vi "Configure Serial Bus (I2S - Trigger).vi"(0 "VISA resource name":refnum<visa-resource-name>, 1 "Data Pattern (0)":string="0", 2 "Lower Threshold (-10)":i32=-10, 5 "Serial Bus Name (1: Serial Bus 1)":i32(ring)=1 items=["Serial Bus 1"=1, "Serial Bus 2"=2], 7 "Trigger Operator (0: Equal)":i32(ring) items=["Equal", "Not Equal", "Less Than", "Greater Than", "In Range", "Out Range", "Increasing", "Decreasing"], 9 "Audio Channel (0: Right Channel)":i32(ring) items=["Right Channel", "Left Channel", "Either"], 11 "error in (no error)":errorcluster, 12 "Pattern Format (0: Binary)":i32(ring) items=["Binary", "Hex", "Decimal"], 13 "Higher Threshold (10)":i32=10) -> (4 "VISA resource name out":refnum<visa-resource-name>, 15 "error out":errorcluster)   [LabVIEW 2017, in "Agilent 2000 3000 X-Series.lvlib"]
doc: "Configures the trigger settings of I2S bus.\n\nNote:\nThis VI is not supported by 1000 X Series"
uses:
  Agilent 2000 3000 X-Series.lvlib
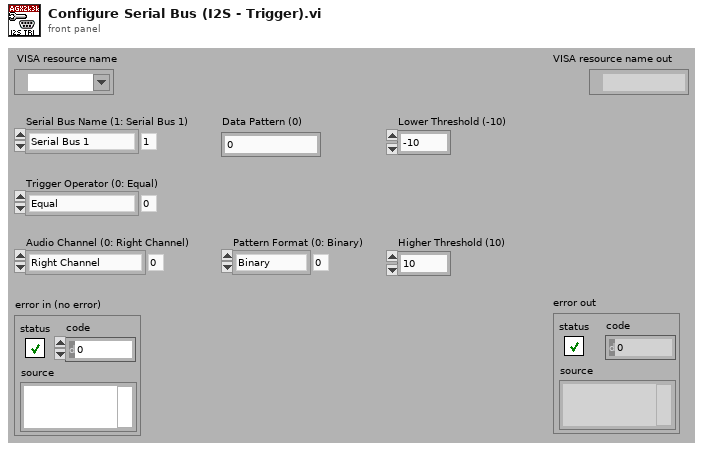
[diagram p1: front panel]
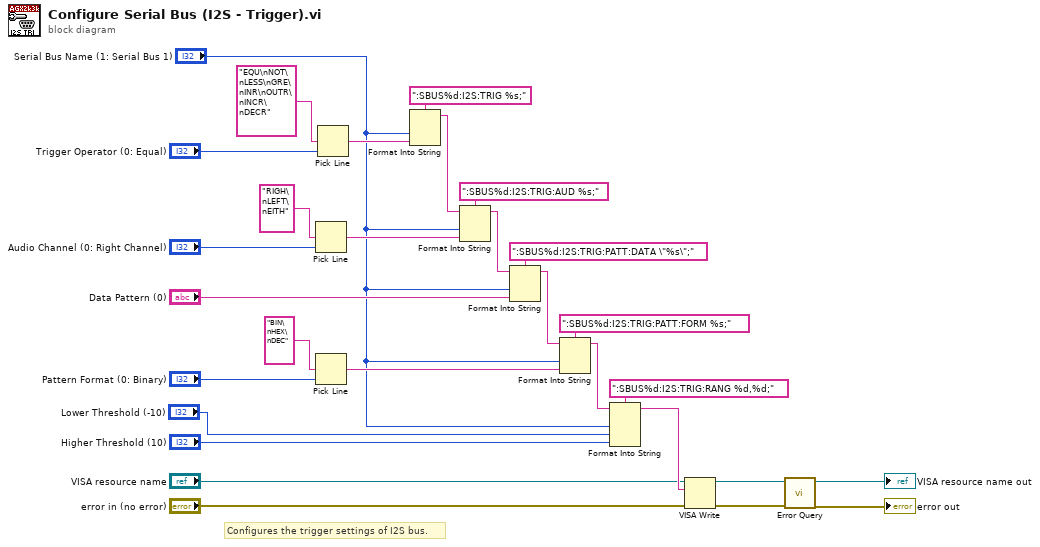
[diagram p0: block diagram]
diagram:
  # "Configures the trigger settings of I2S bus."
  n1 = Pick Line(multi-line string="RIGH\nLEFT\nEITH", line index="Audio Channel (0: Right Channel)") -> (output string=w21:string)  [unwired: 1 out]
  n2 = Pick Line(multi-line string="BIN\nHEX\nDEC", line index="Pattern Format (0: Binary)") -> (output string=w13:string)  [unwired: 1 out]
  n3 = Pick Line(multi-line string="EQU\nNOT\nLESS\nGRE\nINR\nOUTR\nINCR\nDECR", line index="Trigger Operator (0: Equal)") -> (output string=w26:string)  [unwired: 1 out]
  n4 = Format Into String(format string=":SBUS%d:I2S:TRIG %s;", "Serial Bus Name (1: Serial Bus 1)", w26) -> (resulting string=w23:string)  [unwired: 2 in, 1 out]
  n5 = Format Into String(format string=":SBUS%d:I2S:TRIG:AUD %s;", initial string=w23, "Serial Bus Name (1: Serial Bus 1)", w21) -> (resulting string=w20:string)  [unwired: 1 in, 1 out]
  n6 = Format Into String(format string=":SBUS%d:I2S:TRIG:PATT:DATA \"%s\";", initial string=w20, "Serial Bus Name (1: Serial Bus 1)", "Data Pattern (0)") -> (resulting string=w15:string)  [unwired: 1 in, 1 out]
  n7 = Format Into String(format string=":SBUS%d:I2S:TRIG:PATT:FORM %s;", initial string=w15, "Serial Bus Name (1: Serial Bus 1)", w13) -> (resulting string=w12:string)  [unwired: 1 in, 1 out]
  n8 = Format Into String(format string=":SBUS%d:I2S:TRIG:RANG %d,%d;", initial string=w12, "Serial Bus Name (1: Serial Bus 1)", "Lower Threshold (-10)", "Higher Threshold (10)") -> (resulting string=w8:string)  [unwired: 1 in, 1 out]
  n9 = VISA Write(VISA resource name="VISA resource name", write buffer=w8, error in (no error)="error in (no error)") -> (VISA resource name out=w5:refnum<visa-resource-name>, error out=w4:errorcluster)  [unwired: 1 out]
  n10 = call "Error Query.vi"("error in (no error)"=w4, "VISA resource name"=w5) -> ("error out"=→"error out":errorcluster, "VISA resource name out"=→"VISA resource name out":refnum<visa-resource-name>)  [unwired: 8 out]
